vi "01AMT800.vi"() -> ()   [LabVIEW 2015]
uses:
  <vilib>/Utility/error.llb/DialogType.ctl
  <vilib>/Instr/_visa.llb/VISA Configure Serial Port (Serial Instr).vi
panel:
  in  "Tab Control":T1(tab)
  in  "RAMP DOWN":bool
  in  "RAMP UP":bool
  in  "RES DOWN":bool
  in  "RES UP":bool
  out "RAMP":dbl=1.0 min=0.0 max=12.0 step=0.1
  out "RES":dbl=1.0 min=0.0 max=12.0 step=0.1
  out "Reply":string
  out "Error":string
  in  "Command":string
  in  "Insert Command":bool
  in  "Wait":bool
  out "Part":string
  in  "STOP":bool
  in  "Port":refnum<visa-resource-name>
  in  "milliseconds to wait":u32
  out "Data":T2
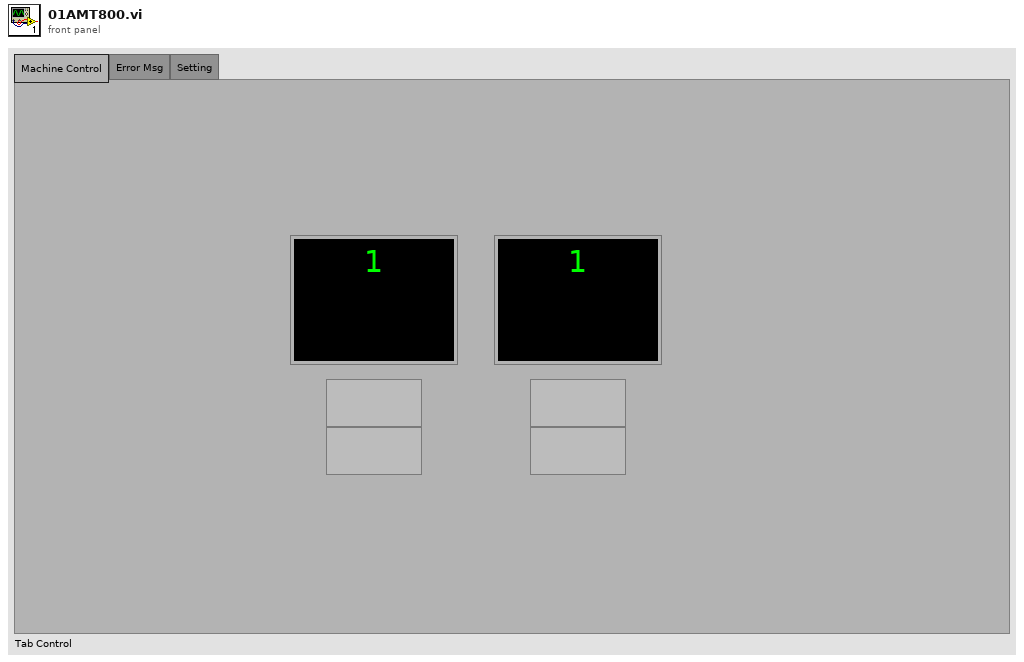
[diagram p1: front panel]
types:
  T1 = enum32{"Machine Control", "Error Msg", "Setting"}
  T2 = cluster{"err":i32[], "vin":i32, "vbus":i32, "amps":i32, "iamp":i32, "mph":i32, "inc":i32, "lift":i32, "vbat":i32}
  T3 = enum16{"Initialize", "Next", "Send RSET", "Set MPH", "Set INC", "Part to 0"}
  T4 = enum16{"err", "mph:", "inc:", "cnfg:", "loop:", "type", "ver", "part:", "led2:", "xmph", "led1", "ptmp", "mtmp", "vbus", "iamp", "vin", "amps", "RSET", "ramp:", "res:", "rng:", "rpm", "vbat", "lift"}[]
  T5 = typedef "DialogType.ctl" = u16
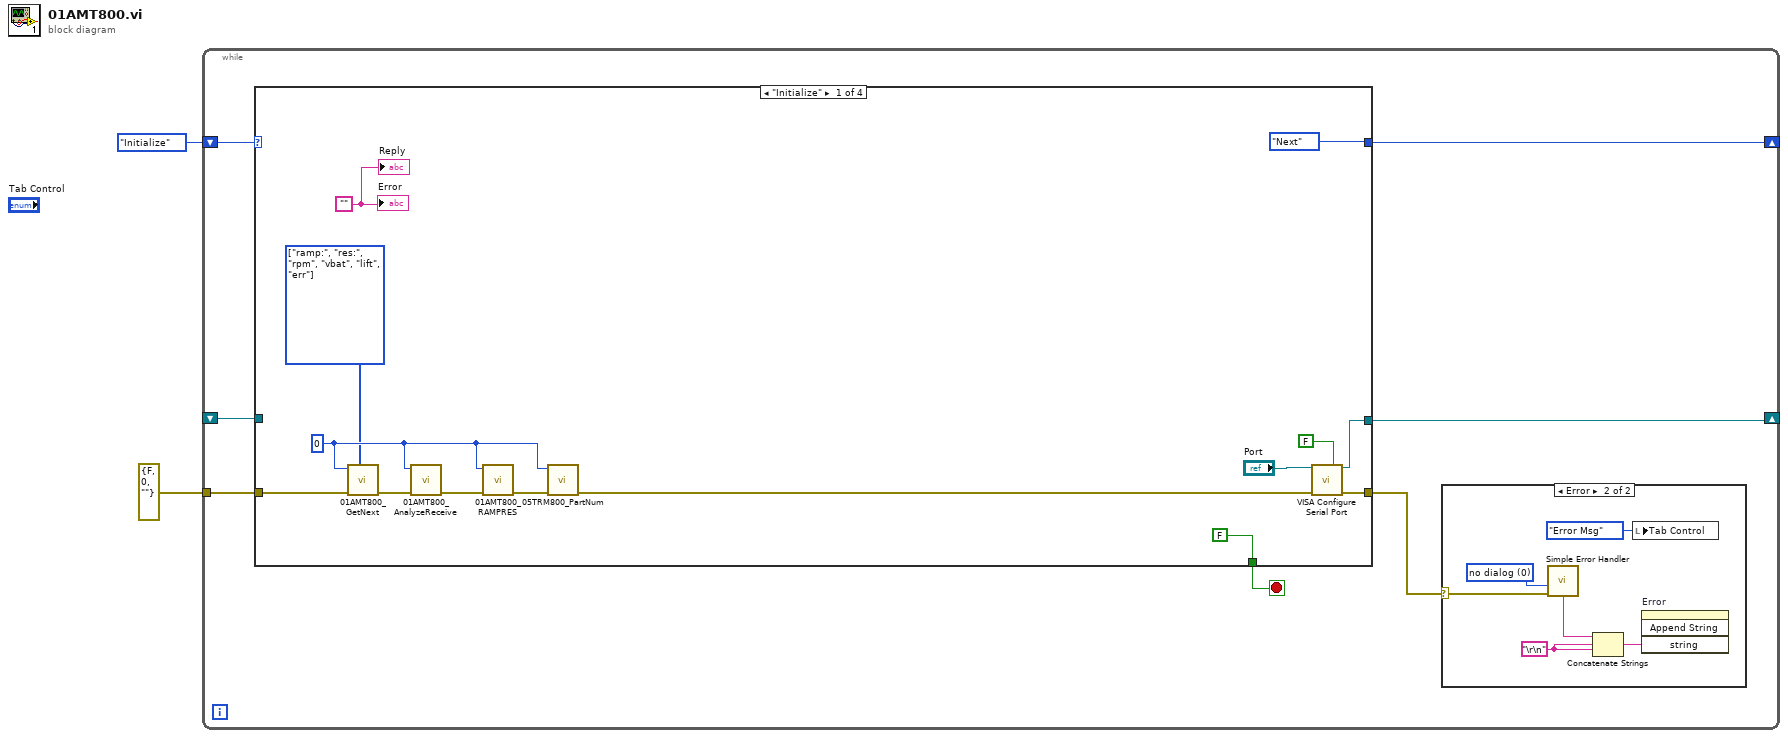
[diagram p0: block diagram]
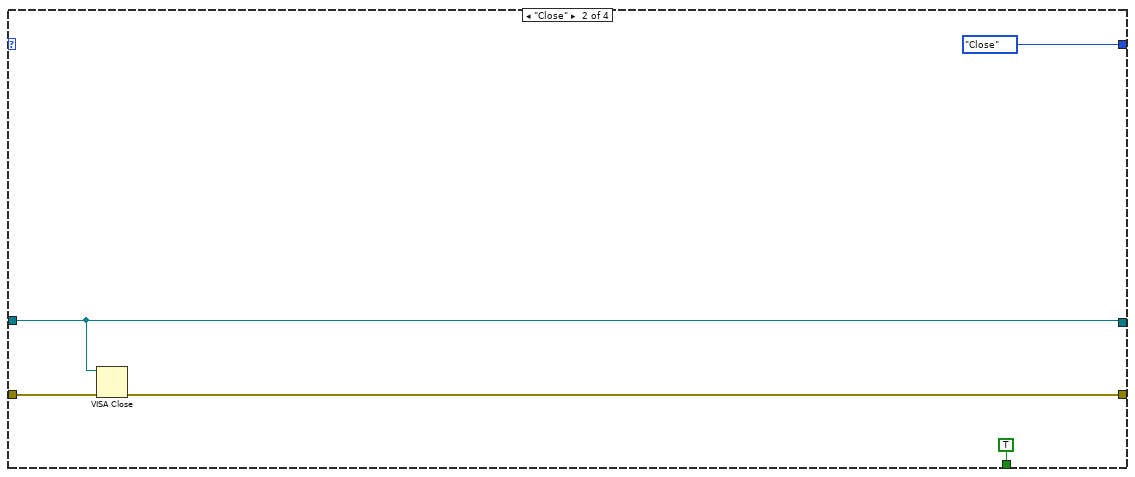
[diagram p3: hidden frame]
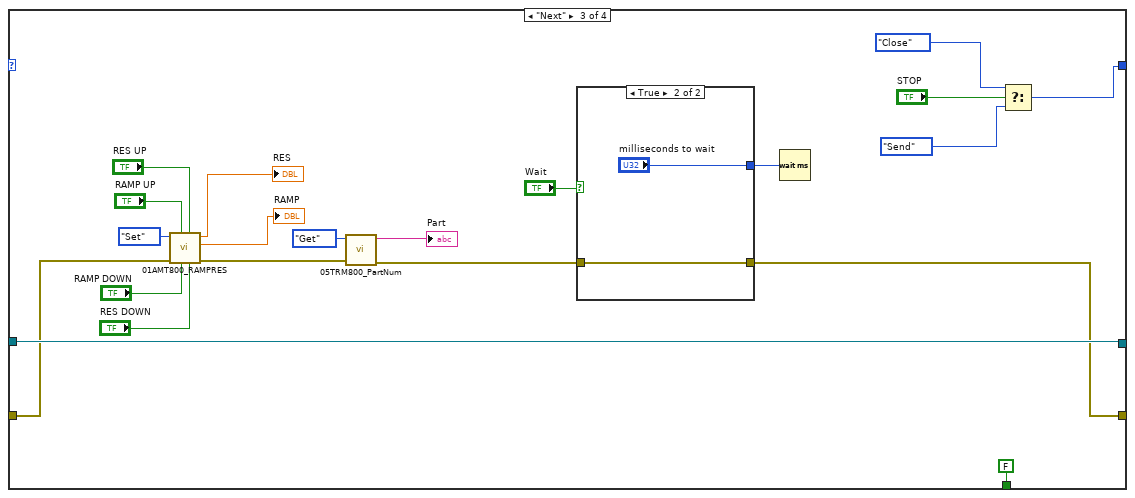
[diagram p4: hidden frame]
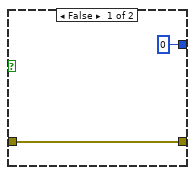
[diagram p5: hidden frame]
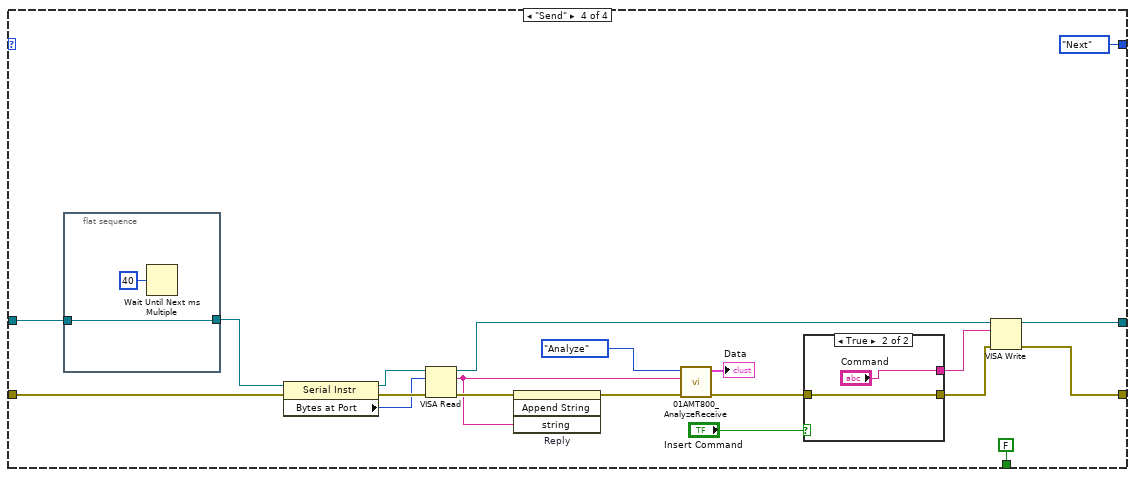
[diagram p6: hidden frame]
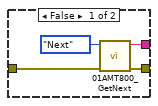
[diagram p7: hidden frame]
diagram:
  n1 = while {
    shift-right: [w8] -> _
    shift-left: enum16{"Initialize", "Close", "Next", "Send"}."Initialize" -> [w9]
    tunnel: errorcluster {"status"=FALSE, "code"=0, "source"=""} ("error constant") -> [w6]
    shift-right: [w4] -> _
    shift-left: _ -> [w3]
    stop <- w7 stop-if-true
    n2 = case shown="\"Initialize\"" w9 {
      tunnel: [enum16{"Initialize", "Close", "Next"}."Next" enum16{"Initialize", "Close"}."Close" w53 enum16{"Initialize", "Close", "Next", "Send"}."Next"] -> w8
      tunnel: [FALSE TRUE FALSE FALSE] -> w7
      tunnel: w6 -> [w22 w32 w48 w77]
      tunnel: [w27 w30 w37 w70] -> w5
      tunnel: [w24 w31 w52 w71] -> w4
      tunnel: w3 -> [_ w31 w52 w79]
      frame "Initialize" {
        w16 = T4 [enum."ramp:", enum."res:", enum."rpm", enum."vbat", enum."lift", enum."err"] items=["err", "mph:", "inc:", "cnfg:", "loop:", "type", "ver", "part:", "led2:", "xmph", "led1", "ptmp", "mtmp", "vbus", "iamp", "vin", "amps", "RSET", "ramp:", "res:", "rng:", "rpm", "vbat", "lift"] ("Pattern")
        w19 = u16 0
        w23 = ""
        n3 = call "01AMT800_GetNext.vi"("Pattern"=w16, "error in (no error)"=w22, "Enum"=w19) -> ("error out"=w21:errorcluster)  [unwired: 7 in, 1 out]
        n4 = call "01AMT800_AnalyzeReceive.vi"("error in (no error)"=w21, "Enum"=w19) -> ("error out"=w20:errorcluster)  [unwired: 8 in, 1 out]
        n5 = call "01AMT800_RAMPRES.vi"("error in (no error)"=w20, "Enum"=w19) -> ("error out"=w18:errorcluster)  [unwired: 7 in, 2 out]
        n6 = call "05TRM800_PartNum.vi"("error in (no error)"=w18, "Enum"=w19) -> ("error out"=w17:errorcluster)  [unwired: 8 in, 1 out]
        n7 = call-poly "VISA Configure Serial Port"("VISA resource name"="Port", "Enable Termination\nChar (T)"=FALSE ("Enable Termination\nChar (T)"), "error in (no error)"=w17) -> ("VISA resource name out"=w24:refnum<visa-resource-name>, "error out"=w27:errorcluster)  [unwired: 11 in]
        "Error" <- w23
        "Reply" <- w23
      }
      frame "Close" {
        n8 = VISA Close(VISA resource name=w31, error in (no error)=w32) -> (error out=w30:errorcluster)
      }
      frame "Next" {
        n9 = call "01AMT800_RAMPRES.vi"("RES DOWN"="RES DOWN", "RES UP"="RES UP", "RAMP DOWN"="RAMP DOWN", "RAMP UP"="RAMP UP", "error in (no error)"=w48, "Enum"=enum16{"Initialize", "Set"}."Set") -> ("error out"=w41:errorcluster, "RAMP"=→"RAMP":dbl, "RES"=→"RES":dbl)  [unwired: 3 in]
        n10 = call "05TRM800_PartNum.vi"("error in (no error)"=w41, "Enum"=enum16{"Initialize", "Get", "Input"}."Get") -> ("error out"=w38:errorcluster, "Part Num"=→"Part":string)  [unwired: 8 in]
        n11 = case shown="True" "Wait" {
          tunnel: w38 -> [w57 w59]
          tunnel: [w57 w59] -> w37
          tunnel: [u32 0 ("milliseconds to wait") "milliseconds to wait"] -> w36
          frame False {
          }
          frame True {
          }
        }
        n12 = Wait (ms)(milliseconds to wait=w36) -> ()  [unwired: 1 out]
        n13 = Select(t=enum16{"Initialize", "Close", "Next", "Send"}."Close", s="STOP", f=enum16{"Initialize", "Close", "Next", "Send"}."Send") -> (s? t:f=w53:enum16{"Initialize", "Close", "Next", "Send"})
      }
      frame "Send" {
        n14 = flat-sequence {
          tunnel: w79 -> [w86]
          tunnel: [w86] -> w78
          frame #0 {
            n15 = Wait Until Next ms Multiple(millisecond multiple=u32 40) -> ()  [unwired: 1 out]
          }
        }
        n16 = property class="Serial Instr"(reference=w78, error in=w77) -> (reference out=w75:refnum<visa-resource-name>, error out=w76:errorcluster, "Bytes at Port"=w74:u32)
        n17 = VISA Read(VISA resource name=w75, byte count=w74, error in (no error)=w76) -> (VISA resource name out=w72:refnum<visa-resource-name>, read buffer=w63:string, error out=w73:errorcluster)  [unwired: 1 out]
        n18 = invoke on="Reply" class="Str" method="Append String"(error in=w73, "string"=w63) -> (error out=w65:errorcluster)  [unwired: 2 in, 3 out]
        n19 = call "01AMT800_AnalyzeReceive.vi"("error in (no error)"=w65, "String"=w63, "Enum"=enum16{"Initialize", "Analyze"}."Analyze") -> ("error out"=w64:errorcluster, "Data"=→"Data":T2)  [unwired: 7 in]
        n20 = case shown="True" "Insert Command" {
          tunnel: [w83 "Command"] -> w67
          tunnel: [w82 w84] -> w66
          tunnel: w64 -> [w81 w84]
          frame False {
            n21 = call "01AMT800_GetNext.vi"("error in (no error)"=w81, "Enum"=T3."Next") -> ("error out"=w82:errorcluster, "String"=w83:string)  [unwired: 8 in]
          }
          frame True {
          }
        }
        n22 = VISA Write(VISA resource name=w72, write buffer=w67, error in (no error)=w66) -> (VISA resource name out=w71:refnum<visa-resource-name>, error out=w70:errorcluster)  [unwired: 1 out]
      }
    }
    n23 = case shown="Error" w5 {
      selector: w5 -> [_ w14]
      frame No Error {
      }
      frame Error {
        w11 = "\r\n"
        w15 = T5 0 items=["no dialog", "OK message", "continue or stop message", "OK message + warnings", "continue/stop + warnings"] ("type of dialog (OK msg:1)")
        n24 = call <vilib>:"Simple Error Handler.vi"("type of dialog (OK msg:1)"=w15, "error in (no error)"=w14) -> ("message"=w12:string)  [unwired: 3 in, 4 out]
        n25 = Concatenate Strings(w12, w11, w11) -> (w13:string)
        n26 = local write "Tab Control"(T1."Error Msg" ("Tab Control")) -> ()
        n27 = invoke on="Error" class="Str" method="Append String"("string"=w13) -> ()  [unwired: 3 in, 4 out]
      }
    }
  }
